vi "test Copy To Smaller Destination.vi"(8 "error in (no error)":errorcluster, 11 "TestCase in":refnum<class "Data Manipulation Tests.lvclass">) -> (0 "error out":errorcluster, 3 "TestCase out":refnum<class "Data Manipulation Tests.lvclass">)   [LabVIEW 2020, in "Memory Manager Tests.lvlib" / "Data Manipulation Tests.lvclass"]
uses:
  Data Manipulation Tests.lvclass
  C:/Program Files/National Instruments/LabVIEW 2027/vi.lib/addons/_JKI Toolkits/VI Tester/TestCase.llb/TestCase.lvclass
  <vilib>/addons/_JKI Toolkits/VI Tester/TestCase.llb/TestCase.lvclass
  Classes/Pointer/Pointer.lvclass
  Classes/Pointer/Write 1D I32.vi
  Classes/Pointer/Read 1D I32.vi
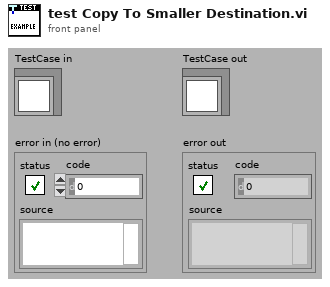
[diagram p1: front panel]
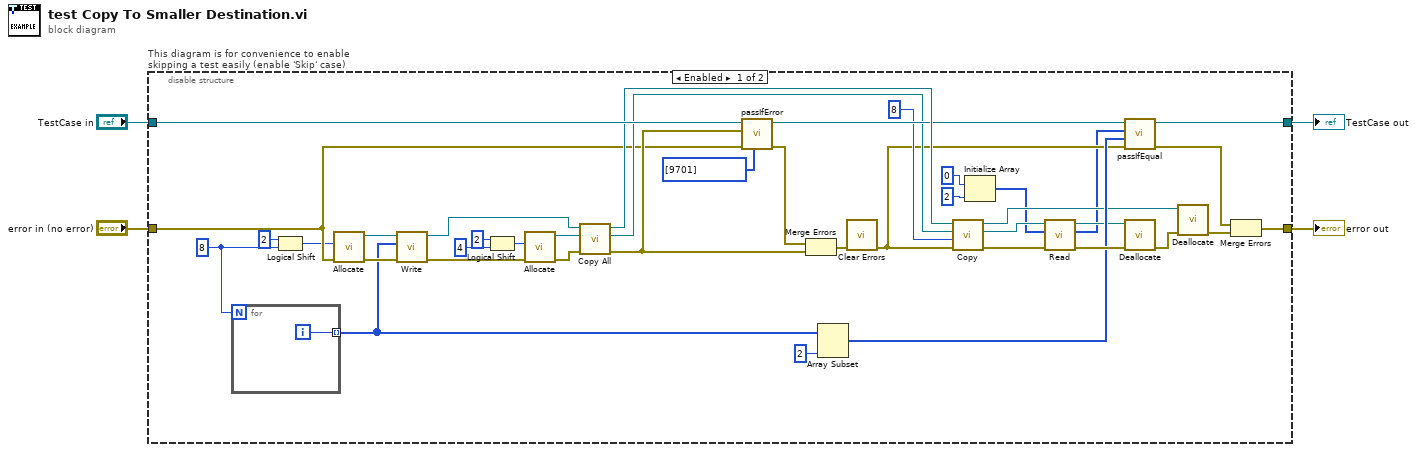
[diagram p0: block diagram]
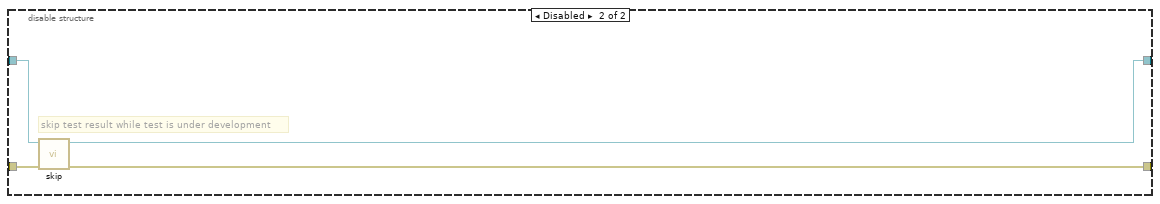
[diagram p2: hidden frame]
diagram:
  n1 = disable-structure "This diagram is for convenience to enable skipping a test easily (enable 'Skip' case)" shown="Enabled" {
    disable-tunnel: "TestCase in" -> [w41 w49]
    disable-tunnel: [w27 w47] -> w1
    disable-tunnel: [w37 w48] -> w3
    disable-tunnel: "error in (no error)" -> [w14 w46]
    frame Enabled {
      w5 = u64 8 ("count (1)")
      n2 = for {
        N: w5 -> [_]
        tunnel: [w45] -> w12 mode=indexing
        i -> [w45]
      }
      n3 = Logical Shift(y=i16 2, x=w5) -> (x << y=w9:u64)
      n4 = call "Allocate.vi"("error in (no error)"=w14, "size"=w9) -> ("error out"=w40:errorcluster, "Pointer out"=w44:refnum<class "Pointer.lvclass">)  [unwired: 8 in]
      n5 = call-poly "Write.vi"("error in (no error)"=w40, "buffer in"=w12, "Pointer in"=w44) -> ("error out"=w39:errorcluster, "Pointer out"=w43:refnum<class "Pointer.lvclass">)  [unwired: 5 in, 2 out]
      n6 = Logical Shift(y=i16 2, x=u64 4 ("count (1)")) -> (x << y=w7:u64)
      n7 = call "Allocate.vi"("error in (no error)"=w39, "size"=w7) -> ("error out"=w38:errorcluster, "Pointer out"=w42:refnum<class "Pointer.lvclass">)  [unwired: 8 in]
      n8 = call "Copy All.vi"("error in (no error)"=w38, "dst Pointer in"=w42, "src Pointer in"=w43) -> ("error out"=w35:errorcluster, "dst Pointer out"=w24:refnum<class "Pointer.lvclass">, "src Pointer out"=w33:refnum<class "Pointer.lvclass">)  [unwired: 6 in]
      n9 = call-dynamic "passIfError.vi"("passing error codes (default = any error code)"=i32[] [9701], "error in (no error)"=w14, "error"=w35, "TestCase in"=w41) -> ("error out"=w16:errorcluster, "TestCase out"=w28:refnum<class "Data Manipulation Tests.lvclass">)  [unwired: 6 in]
      n10 = Merge Errors(w16, w35) -> (w15:errorcluster)
      n11 = Array Subset(array=w12, length=2) -> (w22:i32[])  [unwired: 1 in]
      n12 = call <vilib>:"Clear Errors.vi"("error in (no error)"=w15) -> ("error out"=w13:errorcluster)  [unwired: 5 in, 1 out]
      n13 = call "Copy.vi"("error in (no error)"=w13, "size"=u64 8 ("bytes to copy"), "dst Pointer in"=w24, "src Pointer in"=w33) -> ("error out"=w34:errorcluster, "dst Pointer out"=w31:refnum<class "Pointer.lvclass">, "src Pointer out"=w17:refnum<class "Pointer.lvclass">)  [unwired: 4 in, 1 out]
      n14 = Initialize Array(0 ("Numeric"), 2 ("dimension size")) -> (w11:i32[])
      n15 = call-poly "Read.vi"("error in (no error)"=w34, "buffer in"=w11, "Pointer in"=w31) -> ("error out"=w32:errorcluster, "buffer out"=w10:i32[], "Pointer out"=w19:refnum<class "Pointer.lvclass">)  [unwired: 5 in, 1 out]
      n16 = call-dynamic "passIfEqual.vi"("error in (no error)"=w13, "y"=w22, "x"=w10, "TestCase in"=w28) -> ("error out"=w29:errorcluster, "TestCase out"=w27:refnum<class "Data Manipulation Tests.lvclass">)  [unwired: 6 in]
      n17 = call "Deallocate.vi"("error in (no error)"=w32, "Pointer"=w19) -> ("error out"=w20:errorcluster)  [unwired: 8 in, 1 out]
      n18 = call "Deallocate.vi"("error in (no error)"=w20, "Pointer"=w17) -> ("error out"=w18:errorcluster)  [unwired: 8 in, 1 out]
      n19 = Merge Errors(w29, w18) -> (w37:errorcluster)
    }
    frame Disabled {
      # "skip test result while test is under development"
      n20 = call <vilib>:"skip.vi"("error in (no error)"=w46, "TestCase in"=w49) -> ("error out"=w48:errorcluster, "TestCase out"=w47:refnum<class "Data Manipulation Tests.lvclass">)  [unwired: 8 in]
    }
  }
  "error out" <- w3
  "TestCase out" <- w1
